vi "Chronos TDMS Get Folder.vi"(5 "error in (no error)":errorcluster) -> (1 "error out":errorcluster, 2 "dup path":path)   [LabVIEW 2021]
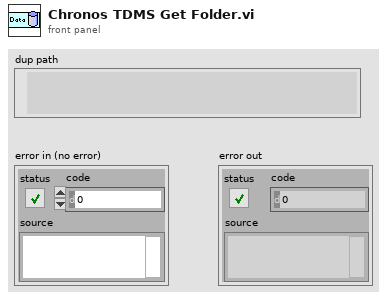
[diagram p1: front panel]
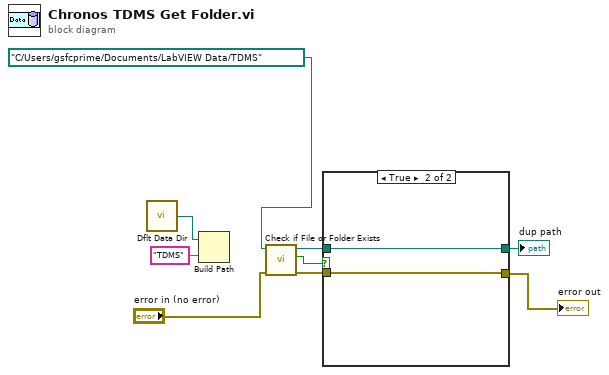
[diagram p0: block diagram]
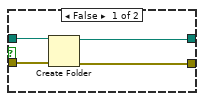
[diagram p2: hidden frame]
diagram:
  n1 = call <vilib>:"Dflt Data Dir.vi"() -> ("App:Default Data Directory"=w9:path)
  n2 = Build Path(base path=w9, name or relative path="TDMS") -> ()  [unwired: 1 out]
  n3 = call <vilib>:"Check if File or Folder Exists.vi"("error in (no error)"="error in (no error)", "path"=path "C:/Users/gsfcprime/Documents/LabVIEW Data/TDMS") -> ("error out"=w3:errorcluster, "file or folder exists?"=w7:bool, "dup path"=w6:path)  [unwired: 7 in]
  n4 = case shown="True" w7 {
    tunnel: w6 -> [w13 w15]
    tunnel: [w12 w15] -> w5
    tunnel: w3 -> [w11 w14]
    tunnel: [w10 w14] -> w2
    frame False {
      n5 = Create Folder(path (use dialog)=w13, error in=w11) -> (created path=w12:path, error out=w10:errorcluster)  [unwired: 1 in, 1 out]
    }
    frame True {
    }
  }
  "error out" <- w2
  "dup path" <- w5
